vi "Floor_Negative.vi"(10 "Baseline U8":u8, 11 "Input Value":u8) -> (3 "Output Value":u8)   [LabVIEW 2014]
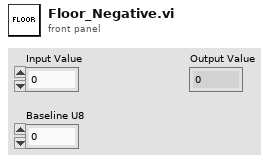
[diagram p1: front panel]
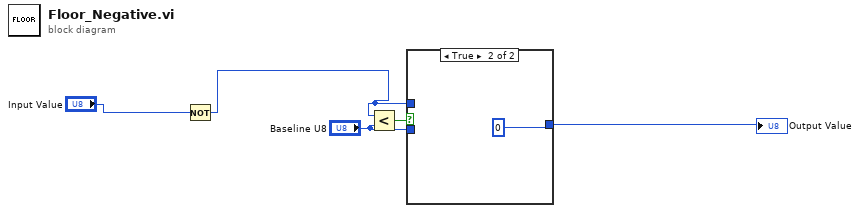
[diagram p0: block diagram]
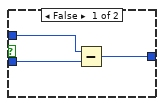
[diagram p2: hidden frame]
diagram:
  n1 = Not(x="Input Value") -> (.not. x?=w1:u8)
  n2 = Less?(x=w1, y="Baseline U8") -> (x < y?=w4:bool)
  n3 = case shown="True" w4 {
    tunnel: w1 -> [w8 _]
    tunnel: "Baseline U8" -> [w7 _]
    tunnel: [w6 u8 0] -> w5
    frame False {
      n4 = Subtract(x=w8, y=w7) -> (x-y=w6:u8)
    }
    frame True {
    }
  }
  "Output Value" <- w5
